vi "PIM IM Order to Base Order.vi"(1 "IM Order":i32) -> (0 "Base Order Index":u8)   [LabVIEW 2011]
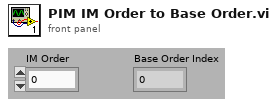
[diagram p1: front panel]
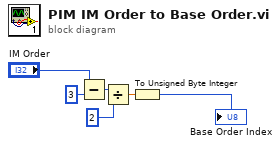
[diagram p0: block diagram]
diagram:
  n1 = Subtract(x="IM Order", y=3 ("index")) -> (x-y=w1:i32)
  n2 = Divide(x=w1, y=2 ("index")) -> (x/y=w2:dbl)
  n3 = To Unsigned Byte Integer(number=w2) -> (unsigned 8bit integer=→"Base Order Index":u8)
